vi "CalculateLegNumRows(SubVI).vi"(8 "Error In":errorcluster, 10 "PlotsNum":dbl, 11 "XYGraph in":refnum<vi>) -> (0 "Error Out":errorcluster, 2 "LegNumRows":dbl, 3 "XYGraph in 2":refnum<vi>)   [LabVIEW 2018]
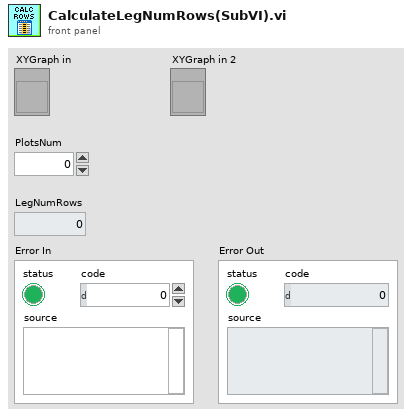
[diagram p1: front panel]
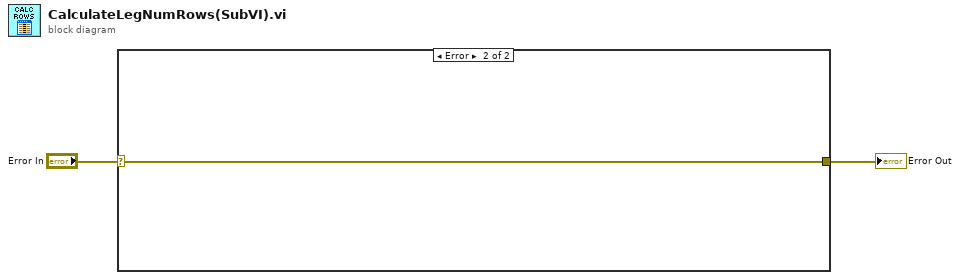
[diagram p0: block diagram]
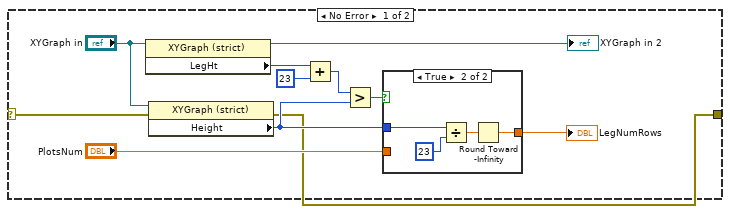
[diagram p2: hidden frame]
diagram:
  n1 = case shown="Error" "Error In" {
    selector: "Error In" -> [w5 w19]
    tunnel: [w4 w19] -> w1
    frame No Error {
      n2 = property on="Property Node" class="XYGraph (strict)"(reference="XYGraph in") -> (reference out=→"XYGraph in 2":refnum<vi>, "LegHt"=w13:u32)  [unwired: 1 in, 1 out]
      n3 = property on="Property Node" class="XYGraph (strict)"(reference="XYGraph in", error in=w5) -> (error out=w4:errorcluster, "Height"=w7:u32)  [unwired: 1 out]
      n4 = Add(x=w13, y=u32 23) -> (x+y=w10:u32)
      n5 = Greater?(x=w10, y=w7) -> (0:w9:bool)
      n6 = case shown="True" w9 {
        tunnel: "PlotsNum" -> [w14 _]
        tunnel: w7 -> [_ w16]
        tunnel: [w14 w15] -> w6
        frame False {
        }
        frame True {
          n7 = Divide(x=w16, y=u32 23) -> (x/y=w18:dbl)
          n8 = Round Toward -Infinity(1:w18) -> (0:w15:dbl)
        }
      }
      "LegNumRows" <- w6
    }
    frame Error {
    }
  }
  "Error Out" <- w1
